vi "Dequeue Local Message.vi"(8 "error in":errorcluster, 11 "Msg queue in":refnum<queue>) -> (0 "error out":errorcluster, 1 "Data":variant, 2 "Message":string, 3 "queue out":refnum<queue>)   [LabVIEW 2021, in "Architecture.lvlib"]
doc: "This VI dequeues a message from a local message queue. Used to enqueue states in a single module state machine. \n\nIf it receives an error In, avoids dequeuing and enqueues a standard error state."
uses:
  Architecture.lvlib
  Typedefs/Message.ctl
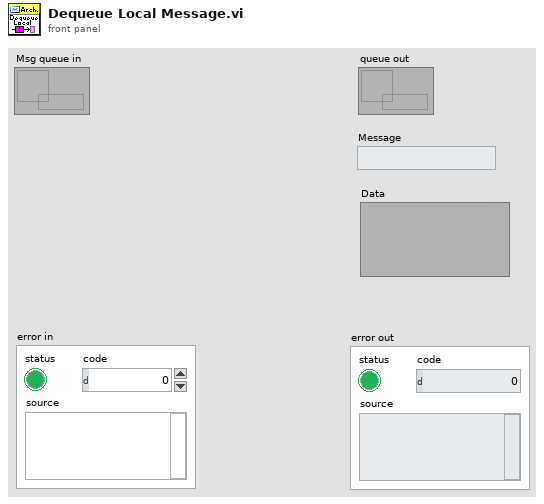
[diagram p1: front panel]
types:
  T1 = typedef "Architecture.lvlib/Message.ctl" = cluster{"Message":string, "Data":variant, "syn":bool}
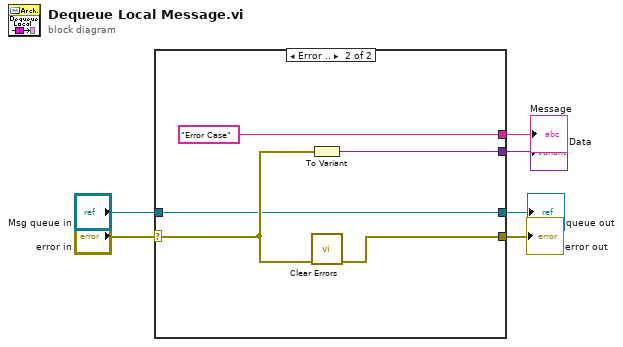
[diagram p0: block diagram]
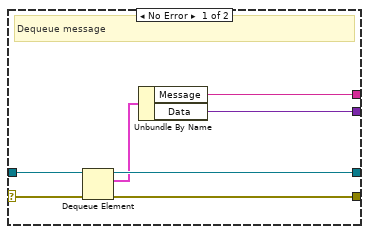
[diagram p2: hidden frame]
diagram:
  n1 = case shown="Error .." "error in" {
    selector: "error in" -> [w12 w18]
    tunnel: "Msg queue in" -> [w13 w16]
    tunnel: [w11 w17] -> w4
    tunnel: [w10 w16] -> w3
    tunnel: [w8 "Error Case" ("Message")] -> w2
    tunnel: [w7 w15] -> w1
    frame No Error {
      # "Dequeue message"
      n2 = Dequeue Element(queue=w13, error in (no error)=w12) -> (queue out=w10:refnum<queue>, element=w9:T1, error out=w11:errorcluster)  [unwired: 1 in, 1 out]
      n3 = Unbundle By Name(w9) -> ("Message"=w8:string, "Data"=w7:variant)
    }
    frame Error {
      n4 = To Variant(anything=w18) -> (Variant=w15:variant)
      n5 = call <vilib>:"Clear Errors.vi"("error in (no error)"=w18) -> ("error out"=w17:errorcluster)  [unwired: 5 in, 1 out]
    }
  }
  "error out" <- w4
  "queue out" <- w3
  "Message" <- w2
  "Data" <- w1
